vi "SGL-to-IEEE754.vi"(11 "Input_DBL":sgl(slide) scale=-20.0..20.0) -> (3 "Output_U8":u8[](array[numeric]))   [LabVIEW 2017]
panel:
  out "*(type *) &x 2":u32
  out "Array":bool[][](array[boolean])
  out "appended array":bool[](array[boolean])
  out "Sign":bool=TRUE
  out "Mantissa":bool[](array[boolean])=[TRUE, FALSE, FALSE, TRUE, FALSE, TRUE, FALSE, FALSE, FALSE, TRUE, TRUE, FALSE, FALSE, TRUE, TRUE, TRUE, FALSE, TRUE, TRUE, FALSE, TRUE, TRUE, FALSE]
  out "Exponent":bool[](array[boolean])=[TRUE, FALSE, FALSE, FALSE, FALSE, TRUE, FALSE, TRUE]
  out "Number":sgl=-101.101 format="%.12f"
  out "Exponent 2":sgl=6.0 format="%.2f"
  out "Mantissa 2":sgl=1.5797031 format="%.8f"
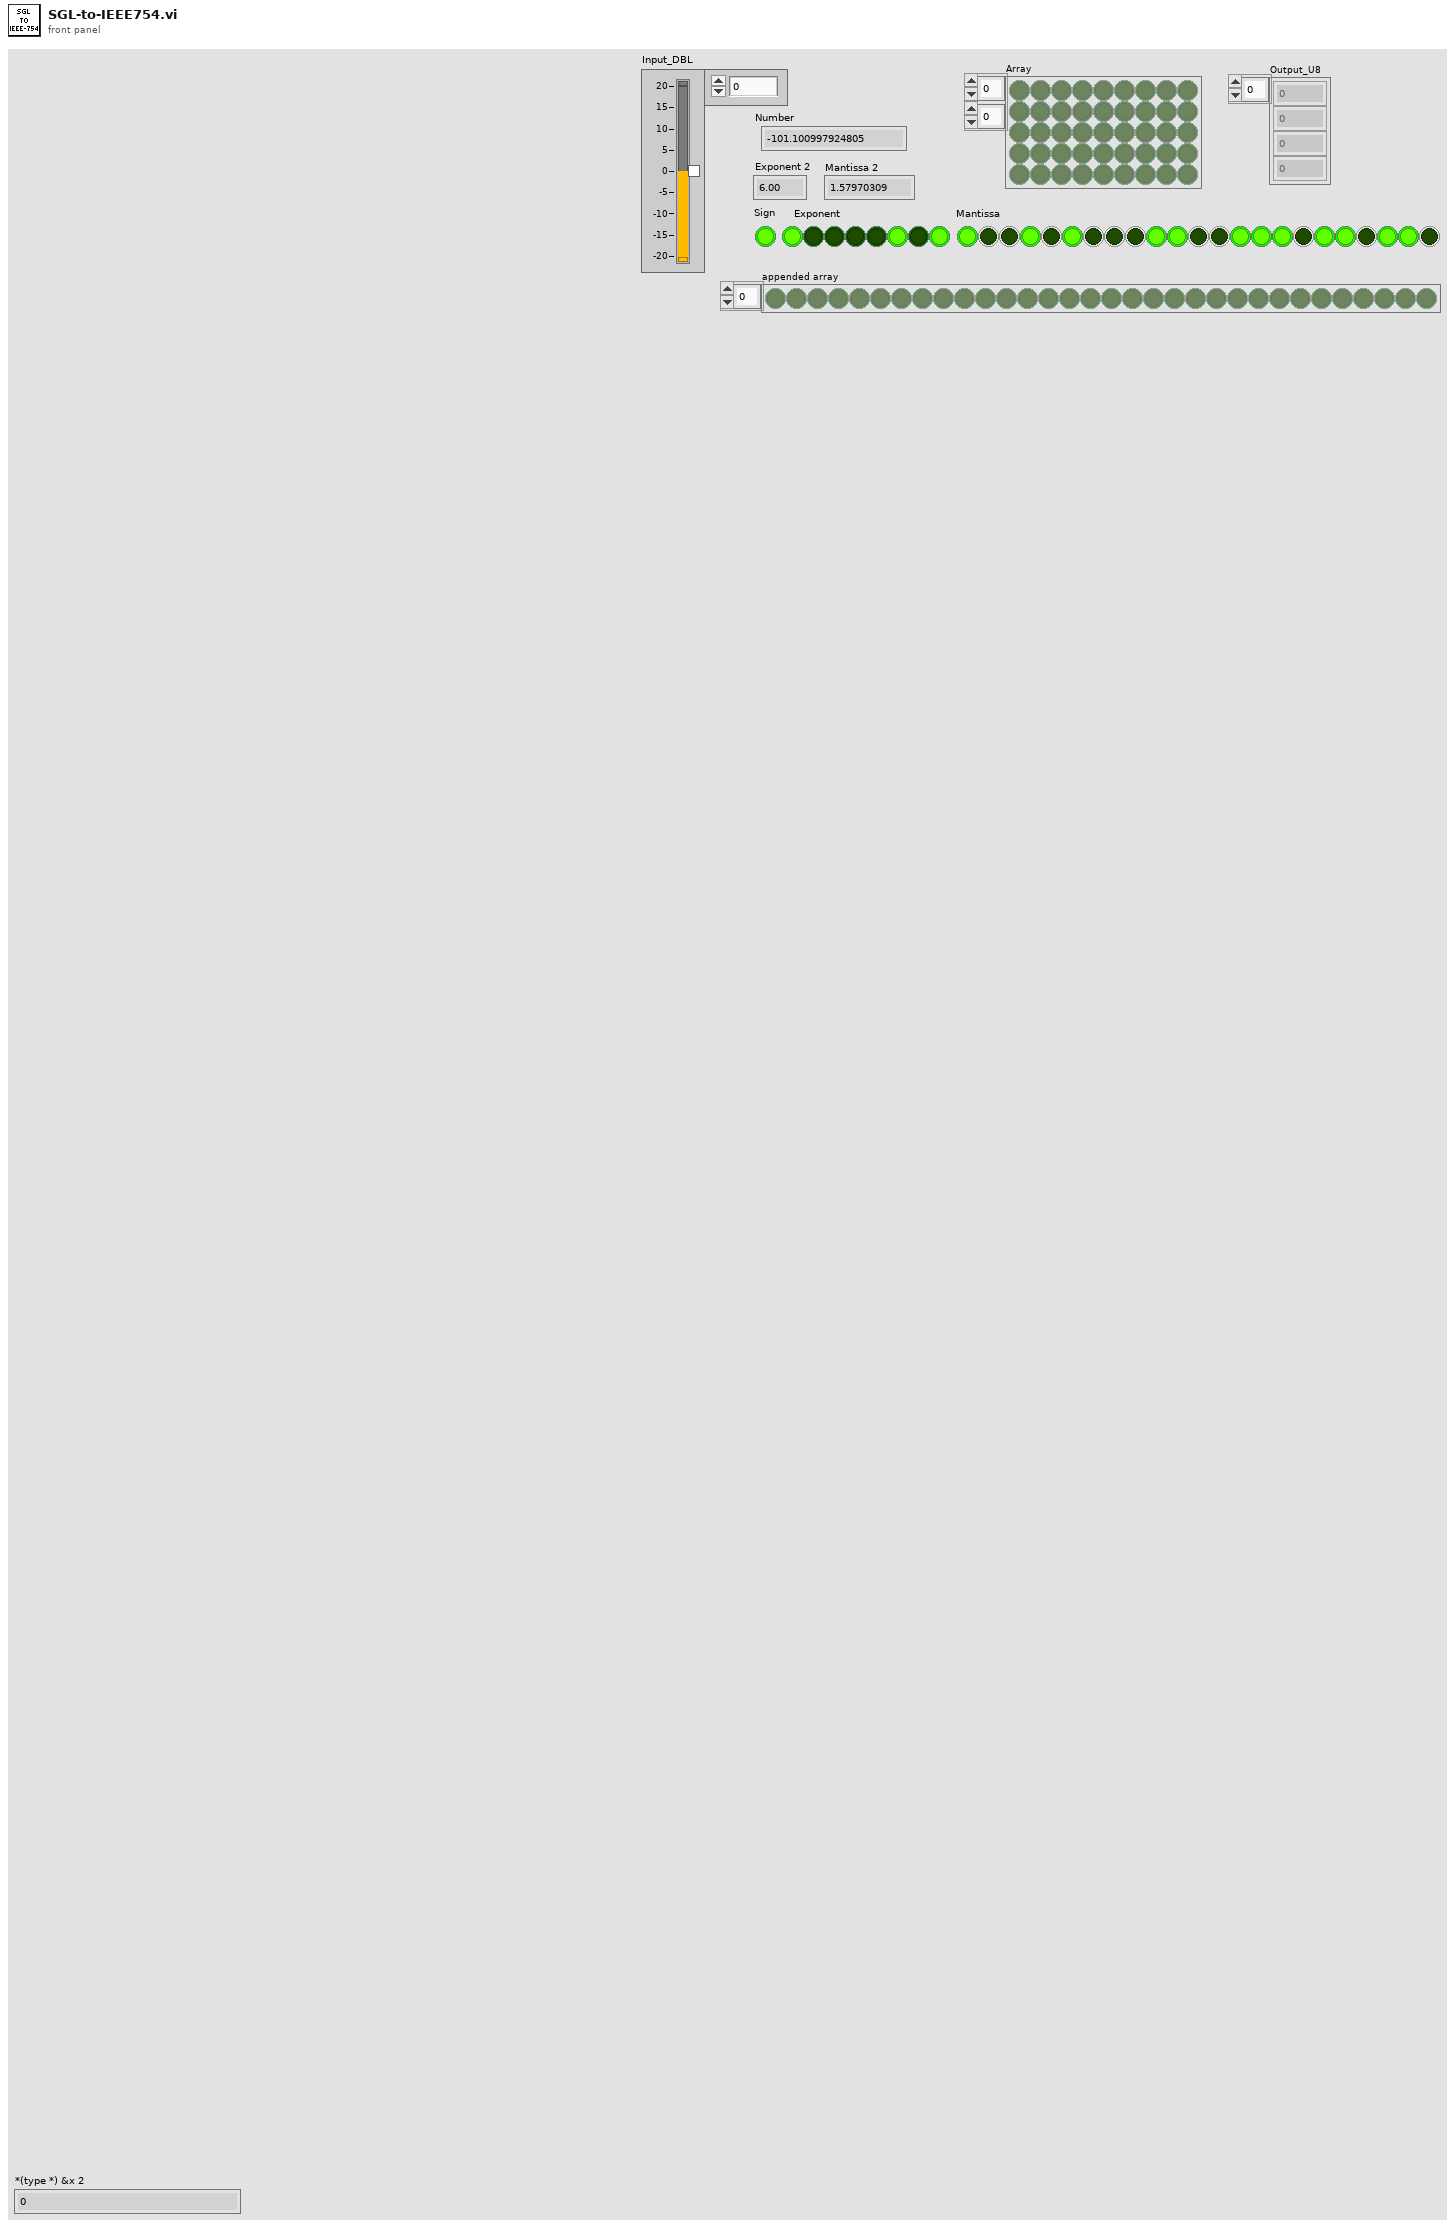
[diagram p1: front panel]
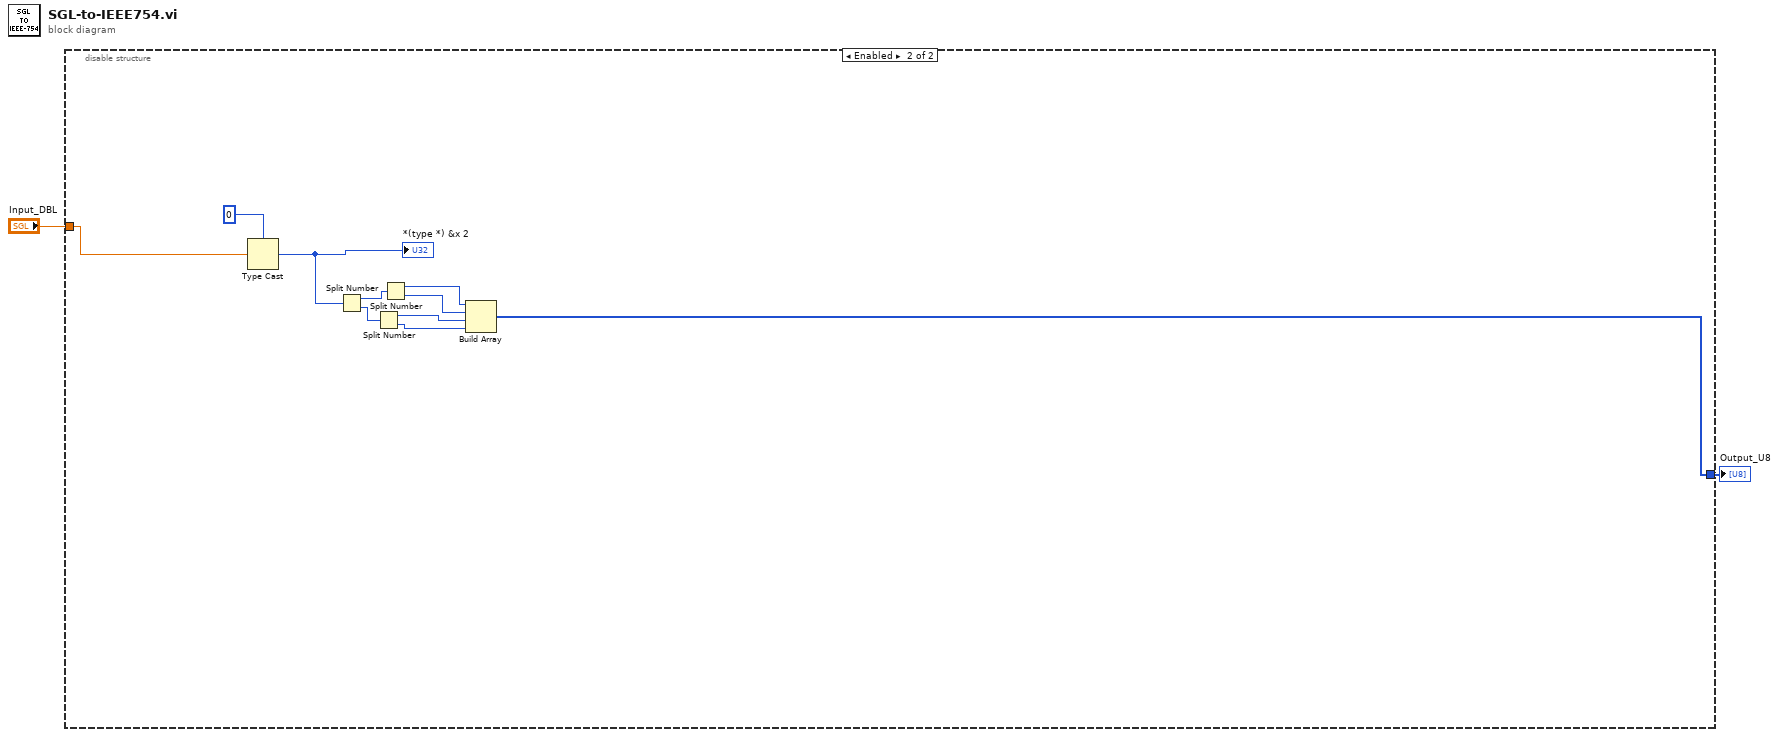
[diagram p0: block diagram]
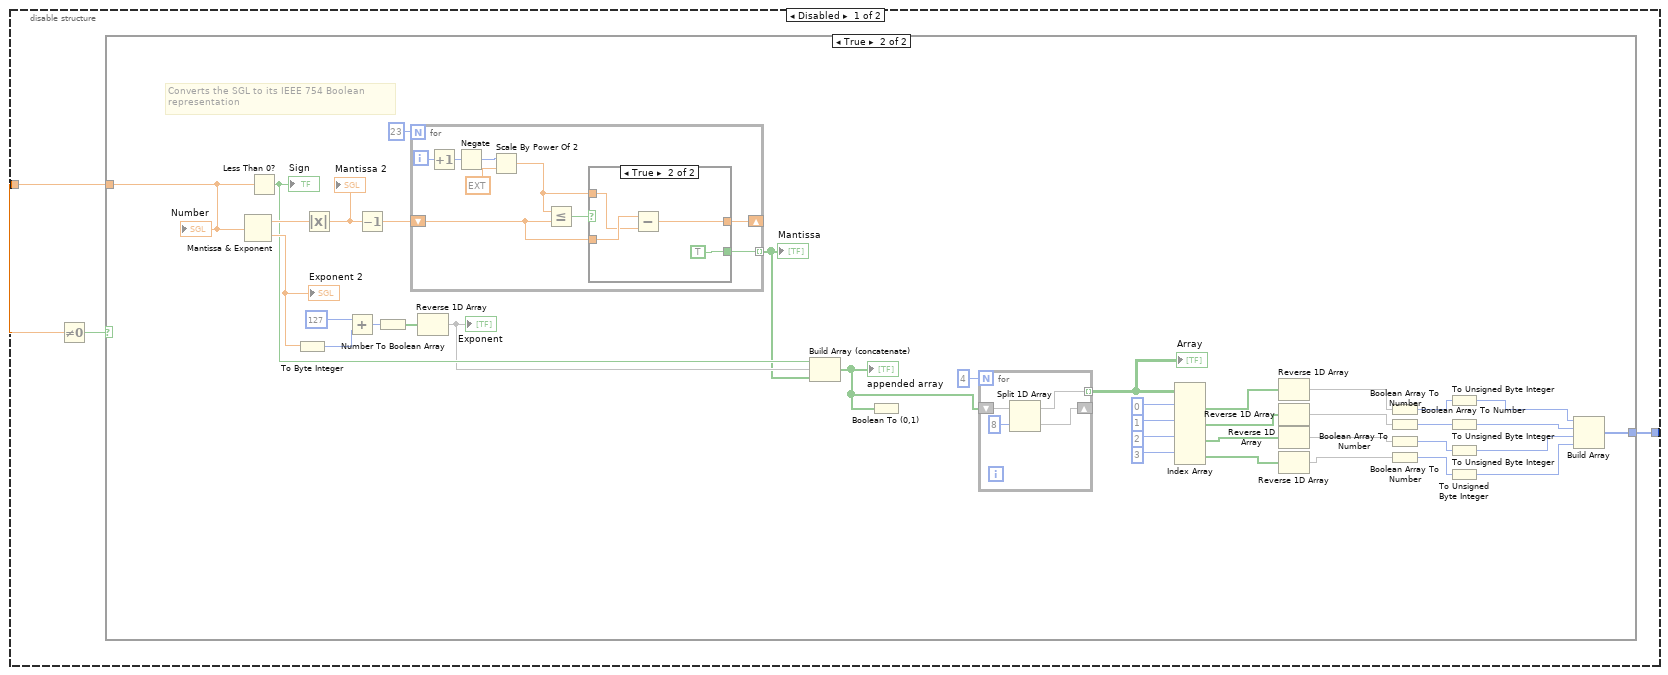
[diagram p2: hidden frame]
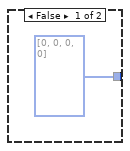
[diagram p3: hidden frame]
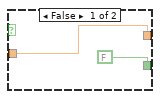
[diagram p4: hidden frame]
diagram:
  n1 = disable-structure shown="Enabled" {
    disable-tunnel: [w5 w63] -> w2
    disable-tunnel: "Input_DBL" -> [w3 w65]
    frame Disabled {
      n2 = Not Equal To 0?(x=w3) -> (x != 0?=w4:bool)
      n3 = case shown="True" w4 {
        tunnel: w3 -> [_ w20]
        tunnel: [u8[] [0, 0, 0, 0] w19] -> w5
        frame False {
        }
        frame True {
          # "Converts the SGL to its IEEE 754 Boolean \nrepresentation"
          n4 = Mantissa & Exponent(0:w20) -> (1:w35:sgl, 2:w37:sgl)
          "Exponent 2" <- w37
          n5 = Less Than 0?(x=w20) -> (x < 0?=w34:bool)
          "Sign" <- w34
          n6 = To Byte Integer(number=w37) -> (8bit integer=w43:i8)
          n7 = Absolute Value(x=w35) -> (abs(x)=w36:sgl)
          "Mantissa 2" <- w36
          n8 = Add(x=i8 127, y=w43) -> (x+y=w42:i8)
          n9 = Decrement(x=w36) -> (x-1=w39:sgl)
          n10 = Number To Boolean Array(number=w42) -> (Boolean array=w41:bool[])
          n11 = for {
            N: 23 -> [_]
            shift-right: [w49] -> _
            shift-left: w39 -> [w51]
            tunnel: [w48] -> w32 mode=indexing
            i -> [w56]
            n12 = Increment(x=w56) -> (x+1=w55:i32)
            n13 = Negate(x=w55) -> (-x=w54:i32)
            n14 = Scale By Power Of 2(n=w54, x=ext 1.0) -> (x*2^n=w50:ext)
            n15 = Less Or Equal?(x=w50, y=w51) -> (x <= y?=w52:bool)
            n16 = case shown="True" w52 {
              tunnel: w51 -> [w57 w62]
              tunnel: w50 -> [_ w59]
              tunnel: [w57 w61] -> w49
              tunnel: [FALSE TRUE] -> w48
              frame False {
              }
              frame True {
                n17 = Subtract(x=w62, y=w59) -> (x-y=w61:ext)
              }
            }
          }
          "Mantissa" <- w32
          n18 = Reverse 1D Array(array=w41) -> (reversed array=w33:bool[])
          "Exponent" <- w33
          n19 = Build Array (concatenate)(w34, w33, w32) -> (w30:bool[])
          "appended array" <- w30
          n20 = Boolean To (0,1)(Boolean=w30) -> ()  [unwired: 1 out]
          n21 = for {
            N: 4 -> [_]
            shift-right: [w46] -> _
            shift-left: w30 -> [w47]
            tunnel: [w45] -> w29 mode=indexing
            n22 = Split 1D Array(array=w47, index=8) -> (first subarray=w45:bool[], second subarray=w46:bool[])
          }
          "Array" <- w29
          n23 = Index Array(array=w29, index (row) #1=0 ("disabled index (col)"), index (row) #2=1 ("index (col)"), index (row) #3=2 ("index (col)"), index (row) #4=3 ("index (col)")) -> (element #1=w14:bool[], element #2=w13:bool[], element #3=w12:bool[], element #4=w11:bool[])  [unwired: 4 in]
          n24 = Reverse 1D Array(array=w14) -> (reversed array=w7:bool[])
          n25 = Reverse 1D Array(array=w13) -> (reversed array=w8:bool[])
          n26 = Reverse 1D Array(array=w12) -> (reversed array=w9:bool[])
          n27 = Reverse 1D Array(array=w11) -> (reversed array=w10:bool[])
          n28 = Boolean Array To Number(Boolean array=w7) -> (number=w24:u32)
          n29 = Boolean Array To Number(Boolean array=w8) -> (number=w23:u32)
          n30 = Boolean Array To Number(Boolean array=w9) -> (number=w22:u32)
          n31 = Boolean Array To Number(Boolean array=w10) -> (number=w21:u32)
          n32 = To Unsigned Byte Integer(number=w24) -> (unsigned 8bit integer=w18:u8)
          n33 = To Unsigned Byte Integer(number=w23) -> (unsigned 8bit integer=w17:u8)
          n34 = To Unsigned Byte Integer(number=w22) -> (unsigned 8bit integer=w16:u8)
          n35 = To Unsigned Byte Integer(number=w21) -> (unsigned 8bit integer=w15:u8)
          n36 = Build Array(w18, w17, w16, w15) -> (w19:u8[])
          "Number" <- w20
        }
      }
    }
    frame Enabled {
      n37 = Type Cast(type=u32 0 ("*(type *) &x 3"), x=w65) -> (*(type *) &x=w66:u32)
      "*(type *) &x 2" <- w66
      n38 = Split Number(x=w66) -> (hi(x)=w67:u16, lo(x)=w68:u16)
      n39 = Split Number(x=w68) -> (hi(x)=w71:u8, lo(x)=w72:u8)
      n40 = Split Number(x=w67) -> (hi(x)=w69:u8, lo(x)=w70:u8)
      n41 = Build Array(w69, w70, w71, w72) -> (w63:u8[])
    }
  }
  "Output_U8" <- w2
